vi "StreamReader Strings.vi"() -> ()   [LabVIEW 2024, in "StreamReader.lvlib" / "StreamReader.lvclass"]
uses:
  StreamReader.lvclass
panel:
  in  "Channel Format String":string="SR%d"
  in  "Reader URL":string="Reader URL"
  in  "Buffer size":string="Buffer size"
  in  "Timeout":string="Timeout"
  in  "Writer URL":string="Writer URL"
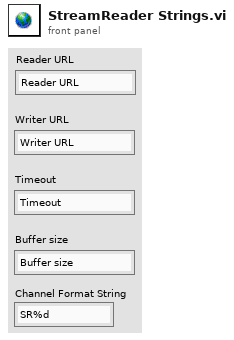
[diagram p1: front panel]
diagram:
